vi "svx_Oct_Build Format String.vi"(1 "trailing zeros":bool, 2 "Precision Type":u16(ring) items=["Digits of precision", "Significant digits"], 3 "Digits":u8, 4 "Type":i32(listbox)) -> (0 "String":string)   [LabVIEW 2017, in "SVX Octave Waterfall Graph.xctl"]
uses:
  <vilib>/addons/_XControls/Octave Waterfall Graph/SVX Octave Waterfall Graph.xctl
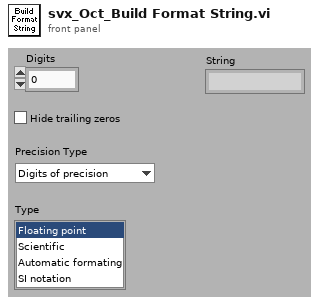
[diagram p1: front panel]
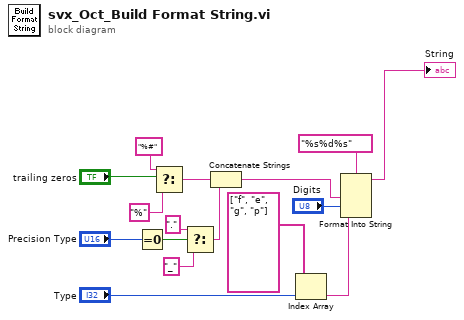
[diagram p0: block diagram]
diagram:
  n1 = Equal To 0?(x="Precision Type") -> (x = 0?=w5:bool)
  n2 = Select(t="%#" ("input 1"), s="trailing zeros", f="%" ("input 1")) -> (s? t:f=w7:string)
  n3 = Select(t="." ("input 1"), s=w5, f="_" ("input 1")) -> (s? t:f=w6:string)
  n4 = Concatenate Strings(w7, w6) -> (w1:string)
  n5 = Index Array(array=string[] ["f", "e", "g", "p"], index="Type") -> (element=w2:string)
  n6 = Format Into String(format string="%s%d%s", w1, "Digits", w2) -> (resulting string=→"String":string)  [unwired: 2 in, 1 out]
